vi "JAUS Set Target Loop GPS.vi"() -> ()   [LabVIEW 2009]
uses:
  JAUS/Support Files/LocalPose.ctl
  JAUS/Support Files/TimeRec.ctl
  <vilib>/Platform/TimedLoop/XDataNode/XDataNode.xnode
  <vilib>/Platform/TimedLoop/XDataNode/loadlvalarms.vi
  <vilib>/Platform/TimedLoop/XDataNode/timing_clust.ctl
  <vilib>/Platform/TimedLoop/XDataNode/nitl_modes.ctl
  <vilib>/Platform/TimedLoop/XDataNode/wakeup.ctl
  Functional Global Variables/Actions for FG's.ctl
  <vilib>/Platform/TimedLoop/XDataNode/XDNodeRunTimeDep.lvlib
panel:
  in  "LocalPose":T1
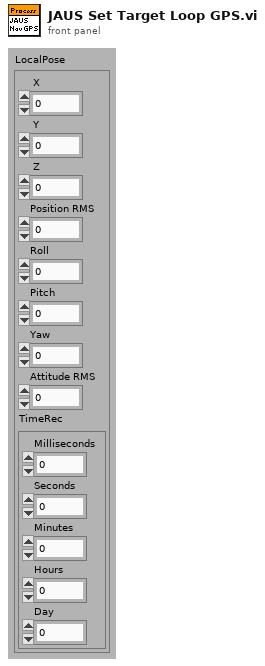
[diagram p1: front panel]
types:
  T1 = typedef "LocalPose.ctl" = cluster{" X":dbl, " Y":dbl, " Z":dbl, "Position RMS":dbl, "Roll":dbl, "Pitch":dbl, "Yaw":dbl, "Attitude RMS":dbl, "TimeRec":T2}
  T2 = typedef "TimeRec.ctl" = cluster{"Milliseconds":u32, "Seconds":u32, "Minutes":u32, "Hours":u32, "Day":u32}
  T3 = typedef "XDNodeRunTimeDep.lvlib/timing_clust.ctl" = cluster{"Expected End [f-1]":u64, "Actual End [f-1]":u64, "Finished Late? [f-1]":bool, "Expected End [i-1]":u64, "Actual End [i-1]":u64, "Finished Late? [i-1]":bool, "Expected Start [i]":u64, "Actual Start [i]":u64, "Expected Start [f]":u64, "Actual Start [f]":u64, "Source Name":string, "Structure Name":string, "Period":i64, "Deadline":i64, "Offset":i64, "Start":i64, "Priority":i32, "Timeout":i32, "Mode":T4, "Wakeup Reason":T5, "Error":errorcluster, "Source Type":string, "Secondary Source Type":string, "Global End Time":u64, "Global Start Time":u64, "Frame Duration":u64, "Iteration Duration":u64, "Assigned CPU":i32, "I/O Scan Engine Mode":u32}
  T4 = typedef "XDNodeRunTimeDep.lvlib/nitl_modes.ctl" = enum32{"No Change", "Process missed periods, maintain original phase", "Discard missed periods, maintain original phase", "Process missed periods, ignore original phase", "Discard missed periods, ignore original phase"}
  T5 = typedef "XDNodeRunTimeDep.lvlib/wakeup.ctl" = enum32{"Normal", "Aborted", "Asynchronous wakeup", "Timing source error", "Timed loop error", "Timeout"}
  T6 = typedef "Actions for FG's.ctl" = enum16{"Read", "Write"}
  T7 = typedef "ElementRec.ctl" = cluster{"ElementUID":u16, " PreviousUID":u16, " NextUID":u16, "LocalWaypointRec":T8}
  T8 = typedef "LocalWaypointRec.ctl" = cluster{"Presence Vector":u8, " X":dbl, " Y":dbl, " Z":dbl, "Roll":dbl, "Pitch":dbl, "Yaw":dbl, "Waypoint Tolerance":dbl, "Path Tolerance":dbl, "Is Active?":bool}
  T9 = typedef "GPS Data.ctl" = cluster{"Latitude":dbl, "Longitude":dbl}
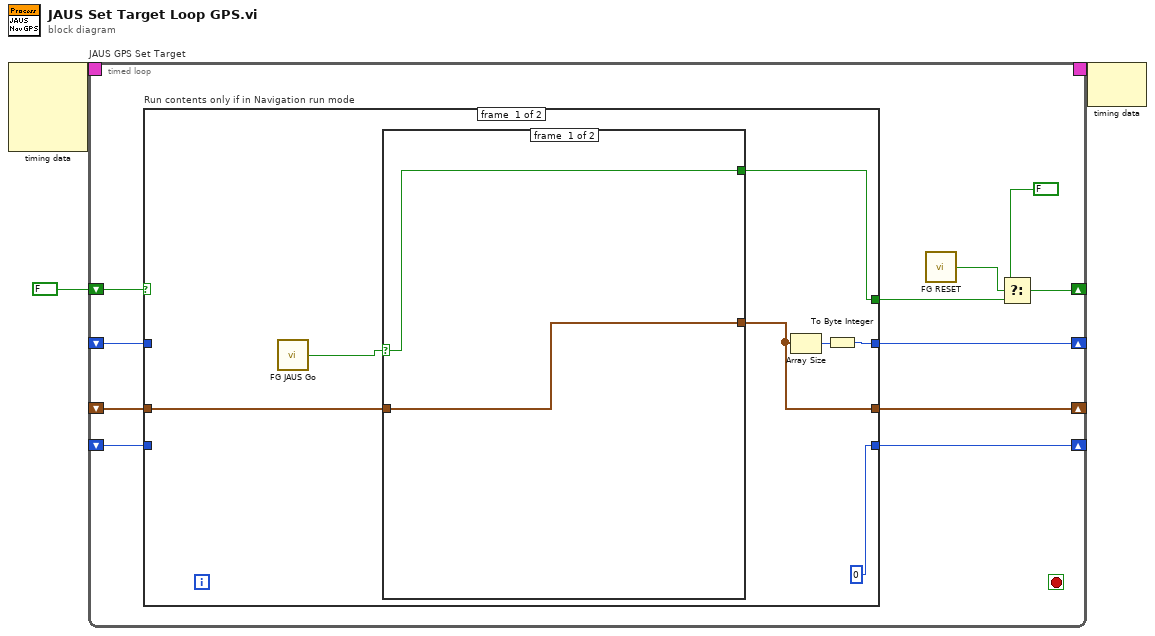
[diagram p0: block diagram]
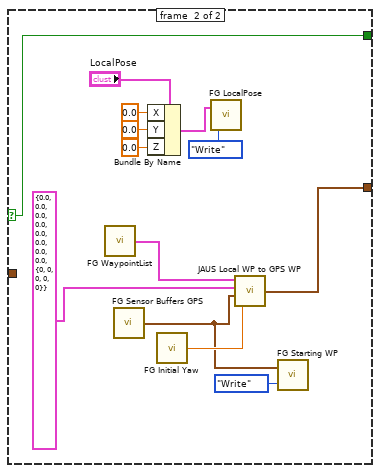
[diagram p2: hidden frame]
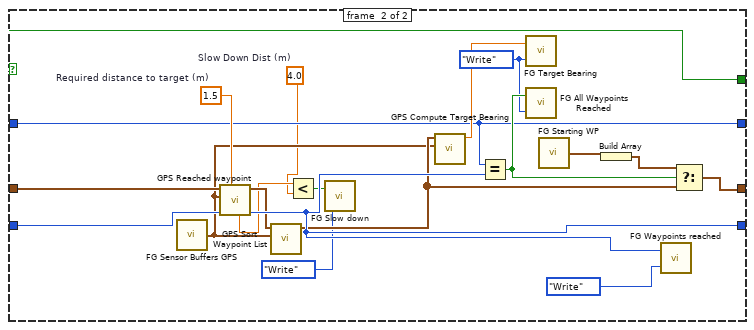
[diagram p3: hidden frame]
diagram:
  n1 = node-c288() -> (w3:T3)  [unwired: 4 in]
  n2 = timed-loop "JAUS GPS Set Target" {
    timing: w3 -> [_]
    timing-out: [_] -> w2
    shift-right: [w12] -> _
    shift-left: _ -> [w14]
    shift-right: [w10] -> _
    shift-left: _ -> [w11]
    shift-right: [w6] -> _
    shift-left: FALSE ("t") -> [w5]
    shift-right: [w9] -> _
    shift-left: _ -> [w13]
    stop <- _ stop-if-true
    n3 = case "Run contents only if in Navigation run mode" shown="False" w5 {
      selector: w5 -> [_ w46]
      tunnel: w14 -> [_ w55]
      tunnel: w13 -> [_ w45]
      tunnel: [i8 0 ("Number of WP Reached OUT") w54] -> w12
      tunnel: w11 -> [w18 w53]
      tunnel: [w16 w49] -> w10
      tunnel: [w21 w46] -> w7
      tunnel: [w19 w45] -> w9
      frame #0 {
        n4 = call "FG JAUS Go.vi"() -> ("Go Out"=w15:bool)  [unwired: 2 in]
        n5 = case shown="True" w15 {
          selector: w15 -> [w23 w36]
          tunnel: [w23 w36] -> w21
          tunnel: w18 -> [w22 _]
          tunnel: [w22 w27] -> w16
          frame #0 {
          }
          frame #1 {
            n6 = call "FG WaypointList.vi"() -> ("Local Waypoint List out"=w29:T7[])  [unwired: 2 in]
            n7 = call "FG Sensor Buffers GPS.vi"() -> ("GPS Buffer out"=w25:T9)  [unwired: 2 in]
            n8 = Bundle By Name(cluster="LocalPose", "X"=0.0, "Y"=0.0, "Z"=0.0) -> (w34:T1)
            n9 = call "FG Initial Yaw.vi"() -> ("Initial Yaw Out"=w28:dbl)  [unwired: 2 in]
            n10 = call "FG LocalPose.vi"("FG Action (Read)"=Actions_for_FG's."Write", "LocalPose in"=w34) -> ()  [unwired: 1 out]
            n11 = call "JAUS Local WP to GPS WP.vi"("Initial Yaw"=w28, "Starting GPS WP"=w25, "LocalPose"=T1 {" X"=0.0, " Y"=0.0, " Z"=0.0, "Position RMS"=0.0, "Roll"=0.0, "Pitch"=0.0, "Yaw"=0.0, "Attitude RMS"=0.0, "TimeRec"={"Milliseconds"=0, "Seconds"=0, "Minutes"=0, "Hours"=0, "Day"=0}}, "Local Waypoint List"=w29) -> ("GPS WP List Out"=w27:T9[])
            n12 = call "FG Starting WP.vi"("FG Action (Read)"=Actions_for_FG's."Write", "Starting WP in"=w25) -> ()  [unwired: 1 out]
          }
        }
        n13 = Array Size(array=w16) -> (size(s)=w20:i32)
        n14 = To Byte Integer(number=w20) -> (8bit integer=w19:i8)
      }
      frame #1 {
        w40 = 4.0  # Slow Down Dist (m)
        w47 = Actions_for_FG's."Write" ("FG Action (Read)")
        w51 = 1.5  # Required distance to target (m)
        n15 = call "FG Sensor Buffers GPS.vi"() -> ("GPS Buffer out"=w42:T9)  [unwired: 2 in]
        n16 = call "GPS Reached waypoint.vi"("Required distance to target (meters)"=w51, "Number of WP Reached IN"=w55, "Current Co-ordinates"=w42, "Waypoint List In"=w53) -> ("Number of WP Reached OUT"=w54:i8, "Waypoint List Out"=w44:T9[], "Distance to Target (meters)"=w41:dbl)  [unwired: 4 in, 1 out]
        n17 = call "GPS Sort Waypoint List.vi"("Current co-ordinate"=w42, "Unsorted Waypoint List"=w44) -> ("Sorted Waypoints"=w43:T9[])  [unwired: 9 in]
        n18 = Less?(x=w41, y=w40) -> (x < y?=w39:bool)
        n19 = call "FG Slow down.vi"("FG Action (Read)"=Actions_for_FG's."Write", "Slow down in"=w39) -> ()  [unwired: 1 out]
        n20 = call "GPS Compute Target Bearing.vi"("Current co-ordinates"=w42, "GPS Waypoint List Out"=w43) -> ("Target Bearing (degrees)"=w56:dbl)  [unwired: 8 in]
        n21 = Equal?(x=w45, y=w54) -> (x = y?=w48:bool)
        n22 = call "FG Target Bearing.vi"("FG Action (Read)"=w47, "Target Bearing in"=w56) -> ()  [unwired: 1 out]
        n23 = call "FG All Waypoints Reached.vi"("FG Action (Read)"=w47, "All waypoints reached in"=w48) -> ()  [unwired: 1 in, 1 out]
        n24 = call "FG Starting WP.vi"() -> ("Starting WP out"=w37:T9)  [unwired: 2 in]
        n25 = Build Array(w37) -> (w50:T9[])
        n26 = call "FG Waypoints reached.vi"("FG Action (Read)"=Actions_for_FG's."Write", "Waypoints reached in"=w54) -> ()  [unwired: 1 in, 1 out]
        n27 = Select(t=w50, s=w48, f=w43) -> (s? t:f=w49:T9[])
      }
    }
    n28 = call "FG RESET.vi"() -> ("RESET out"=w4:bool)  [unwired: 2 in]
    n29 = Select(t=FALSE, s=w4, f=w7) -> (s? t:f=w6:bool)
  }
  n30 = node-c288(w2) -> ()  [unwired: 1 out]
